vi "dsf config file target name.vi"() -> (3 "config file target name":string)   [LabVIEW 2020, in "DSF Shared.lvlib"]
uses:
  DSF Shared.lvlib
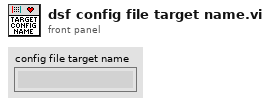
[diagram p1: front panel]
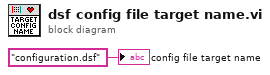
[diagram p0: block diagram]
diagram:
  "config file target name" <- "configuration.dsf" ("Property Name")
